vi "AutoFeedForwardConversion.vi"(2 "Planned Rotational Velocity (deg/s)":dbl, 3 "Planned Ground Velocity (in/s)":dbl) -> (0 "Equivalent Rotation Joystick Command (ul)":dbl, 1 "Equivalent Strafe Joystick Command (ul)":dbl)   [LabVIEW 2023]
doc: "Converts the feed-forward ground velocity from inches/sec to a unitless drive command and the feed-forward rotational velocity from degrees/sec to a unitless drive command. This VI is intended for use with the FRC 4265 Autonomous Path Planner and the pure-pursuit algorithm."
uses:
  GlobalDrivebase.vi
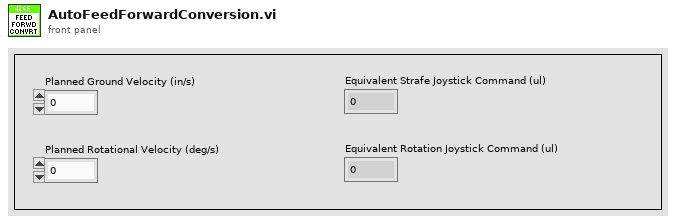
[diagram p1: front panel]
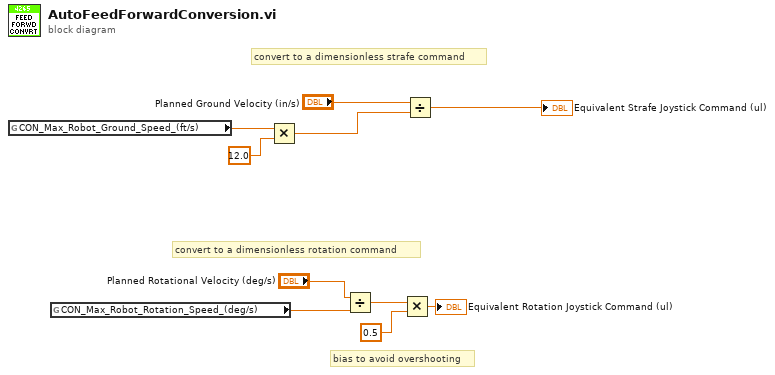
[diagram p0: block diagram]
diagram:
  # "bias to avoid overshooting"
  # "convert to a dimensionless rotation command"
  # "convert to a dimensionless strafe command"
  n1 = global read "GlobalDrivebase.vi" "CON_Max_Robot_Ground_Speed_(ft/s)"() -> (w3:dbl)
  n2 = global read "GlobalDrivebase.vi" "CON_Max_Robot_Rotation_Speed_(deg/s)"() -> (w2:dbl)
  n3 = Multiply(x=w3, y=12.0) -> (x*y=w9:dbl)
  n4 = Divide(x="Planned Rotational Velocity (deg/s)", y=w2) -> (x/y=w5:dbl)
  n5 = Multiply(x=w5, y=0.5 ("Rotation Feed Forward Suppression")) -> (x*y=→"Equivalent Rotation Joystick Command (ul)":dbl)
  n6 = Divide(x="Planned Ground Velocity (in/s)", y=w9) -> (x/y=→"Equivalent Strafe Joystick Command (ul)":dbl)
